vi "PP.GUI.vi"() -> ()   [LabVIEW 2020, in "PixPack.lvlib"]
uses:
  PixPack.lvlib
  12606764-d785-45b7-9cb2-a71dfbc87bf6.vi
  348e77aa-2851-4939-9642-feb7372d7947.vi
  e04cd5c4-3a67-4784-a041-1bf902e3deef.vi
  05c6187d-1229-47b1-81d4-3979da293e79.vi
  d56c83b1-63d8-4632-9ccd-666959e94da8.vi
panel:
  in  "Clear Error":bool
  in  "Password":string
  out "Done":bool
  out "Error":string
  in  "Decode":bool
  in  "Payload File Folder Path [ decode ]":path
  out "error out":errorcluster
  in  "error in":errorcluster
  in  "Encode":bool
  in  "Payload File Path [ encode ]":path
  in  "PNG Path":path
  # "Encode | Decode PNG"
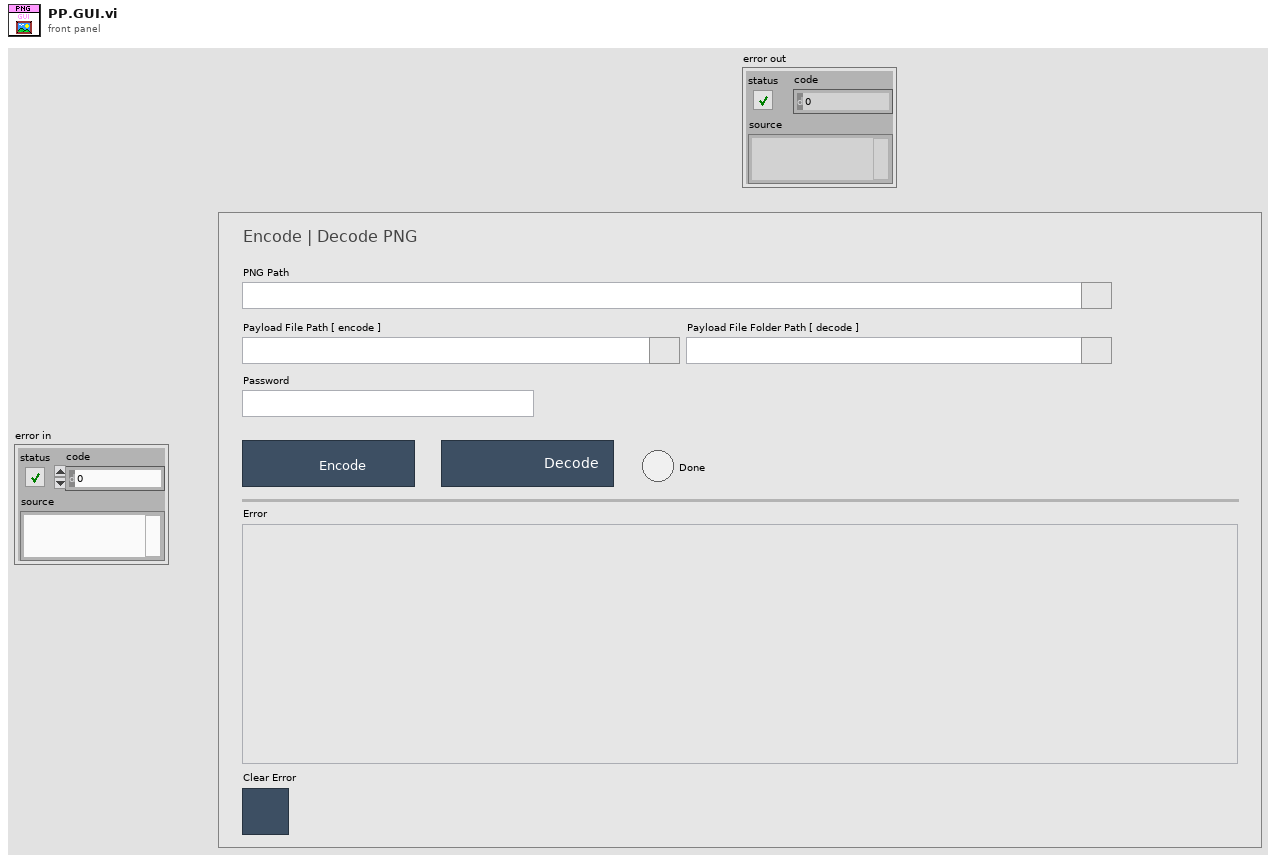
[diagram p1: front panel]
types:
  T1 = enum32{"invalid app kind", "Development System", "Run Time System", "Student Edition", "Embedded LabVIEW", "Evaluation", "Custom"}
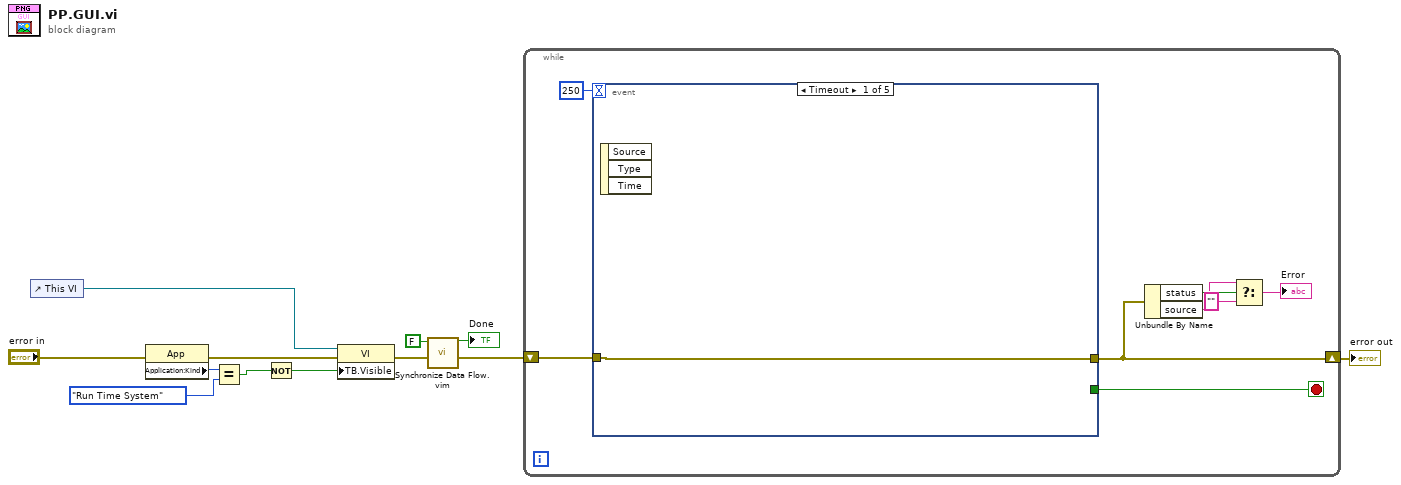
[diagram p0: block diagram]
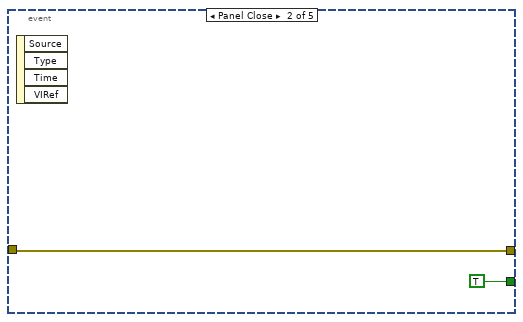
[diagram p2: hidden frame]
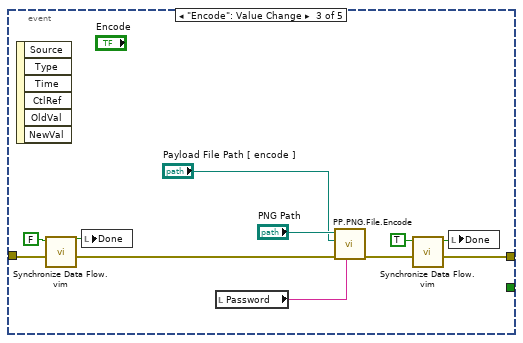
[diagram p3: hidden frame]
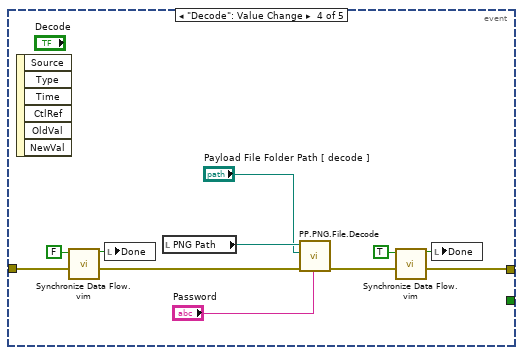
[diagram p4: hidden frame]
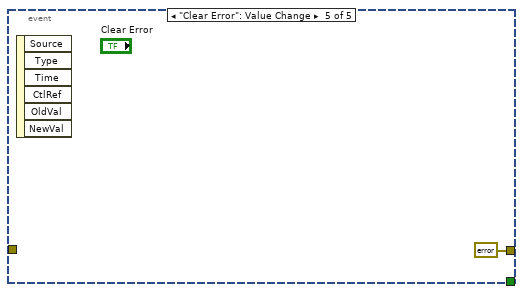
[diagram p5: hidden frame]
diagram:
  n1 = control-ref of="This VI"() -> (w11:refnum<vi>)
  n2 = property class="App"(error in="error in") -> (error out=w7:errorcluster, "Application:Kind"=w9:T1)  [unwired: 1 in, 1 out]
  n3 = Equal?(x=w9, y=T1."Run Time System" ("Application:Kind")) -> (x = y?=w6:bool)
  n4 = Not(x=w6) -> (.not. x?=w5:bool)
  n5 = property class="VI"(reference=w11, error in=w7, "TB.Visible"=w5) -> (error out=w3:errorcluster)  [unwired: 1 out]
  n6 = call "Synchronize Data Flow.vim"("input 3"=w3, "input 1"=FALSE) -> ("output 3"=w2:errorcluster, "output 1"=→"Done":bool)  [unwired: 2 in, 2 out]
  n7 = while {
    shift-right: [w17] -> w12
    shift-left: w2 -> [w18]
    stop <- w19 stop-if-true
    n8 = event shown="[0] Timeout" {
      selector: _ -> [_ _ _ _ _]
      dyn-events: _ -> [_ _ _ _ _]
      timeout: 250 -> [_ _ _ _ _]
      tunnel: [_ TRUE _ _ _] -> w19
      tunnel: w18 -> [w21 w22 w29 w43 _]
      tunnel: [w21 w22 w34 w40 errorcluster {"status"=FALSE, "code"=0, "source"=""} ("output 3")] -> w17
      event Timeout {
        n9 = event-data() -> ()  [unwired: 1 in, 3 out]
      }
      event Panel Close {
        n10 = event-data() -> ()  [unwired: 1 in, 4 out]
      }
      event "Encode": Value Change {
        n11 = event-data() -> ()  [unwired: 1 in, 6 out]
        n12 = call "Synchronize Data Flow.vim"("input 3"=w29, "input 1"=FALSE) -> ("output 3"=w28:errorcluster, "output 1"=w30:bool)  [unwired: 2 in, 2 out]
        n13 = local write "Done"(w30) -> ()
        n14 = local read "Password"() -> (w27:string)
        n15 = call "PP.PNG.File.Encode.vi"("Password"=w27, "error in"=w28, "File Path"="Payload File Path [ encode ]", "PNG In"="PNG Path") -> ("error out"=w24:errorcluster)  [unwired: 6 in]
        n16 = call "Synchronize Data Flow.vim"("input 3"=w24, "input 1"=TRUE) -> ("output 3"=w34:errorcluster, "output 1"=w33:bool)  [unwired: 2 in, 2 out]
        n17 = local write "Done"(w33) -> ()
      }
      event "Decode": Value Change {
        n18 = event-data() -> ()  [unwired: 1 in, 6 out]
        n19 = call "Synchronize Data Flow.vim"("input 3"=w43, "input 1"=FALSE) -> ("output 3"=w39:errorcluster, "output 1"=w45:bool)  [unwired: 2 in, 2 out]
        n20 = local write "Done"(w45) -> ()
        n21 = local read "PNG Path"() -> (w37:path)
        n22 = call "PP.PNG.File.Decode.vi"("Password"="Password", "error in"=w39, "File Folder Out"="Payload File Folder Path [ decode ]", "PNG In"=w37) -> ("error out"=w38:errorcluster)  [unwired: 6 in]
        n23 = call "Synchronize Data Flow.vim"("input 3"=w38, "input 1"=TRUE) -> ("output 3"=w40:errorcluster, "output 1"=w41:bool)  [unwired: 2 in, 2 out]
        n24 = local write "Done"(w41) -> ()
      }
      event "Clear Error": Value Change {
        n25 = event-data() -> ()  [unwired: 1 in, 6 out]
      }
    }
    n26 = Unbundle By Name(w17) -> ("status"=w16:bool, "source"=w15:string)
    n27 = Select(t=w15, s=w16, f="") -> (s? t:f=→"Error":string)
  }
  "error out" <- w12
